vi "Read Temperature.vi"   [LabVIEW 2013, in "LVH-Nest.lvlib"]
uses:
  LVH-Nest.lvlib
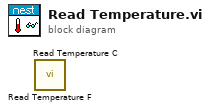
[diagram p0: block diagram]
diagram:
  n1 = call "Read Temperature F.vi"() -> ()  [unwired: 9 in, 3 out]
  n2 = call "Read Temperature C.vi"() -> ()  [unwired: 9 in, 3 out]
